vi "Eurotherm3504_Display.vi"() -> ()   [LabVIEW 2016]
uses:
  TGA_Furnace_v210820.llb/Eurotherm_3504_FP.ctl
panel:
  in  "Eurotherm_3504":T1 {"OP" format="%.2f"; "SP" format="%.1f"; "PV" format="%.1f"}
  # "Ack"
  # "Mode"
  # "Eurotherm"
  # "3504"
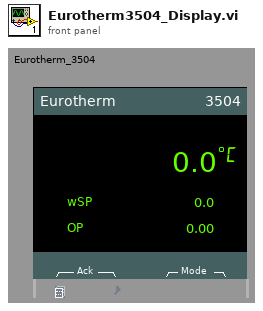
[diagram p1: front panel]
types:
  T1 = typedef "Eurotherm_3504_FP.ctl" = cluster{"PV":dbl, "SP":dbl, "OP":dbl}
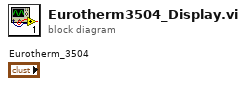
[diagram p0: block diagram]
diagram:
